vi "Parallel Mode Read.vi"(8 "error in":errorcluster, 11 "Cycler in":refnum<class "Cycler.lvclass">) -> (0 "error out":errorcluster, 1 "Changed or First Call?":bool, 2 "Parallel Mode ACT":bool, 3 "Cycler out":refnum<class "Cycler.lvclass">)   [LabVIEW 2023, in "Cycler.lvclass"]
uses:
  Cycler.lvclass
  Low Level Capabilities/Parallel Mode/Parallel Mode.lvclass
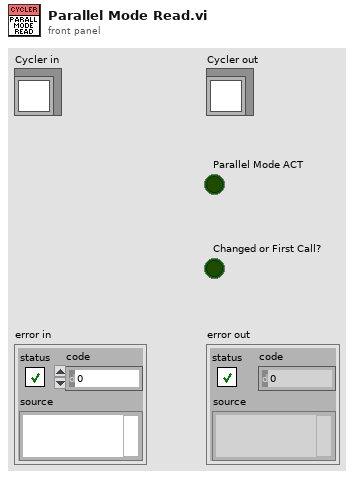
[diagram p1: front panel]
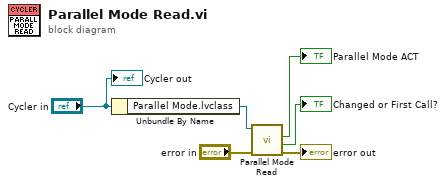
[diagram p0: block diagram]
diagram:
  n1 = Unbundle By Name("Cycler in") -> ("Parallel Mode.lvclass"=w5:refnum<class "Parallel Mode.lvclass">)
  n2 = call-dynamic "Parallel Mode Read.vi"("error in"="error in", "Parallel Mode in"=w5) -> ("error out"=→"error out":errorcluster, "Changed or First Call?"=→"Changed or First Call?":bool, "Parallel Mode ACT"=→"Parallel Mode ACT":bool)  [unwired: 6 in, 1 out]
  "Cycler out" <- "Cycler in"
